vi "test_AllCodeInCorrectLVVersion.vi"() -> (3 "Pass?":bool)   [LabVIEW 2019, in "Tests.General.lvlib"]
uses:
  Tests.General.lvlib
panel:
  in  "LV version":string="19.0"
  out "Failed results":cluster{"file":path, "FileLVVersion":string}[](array[cluster])
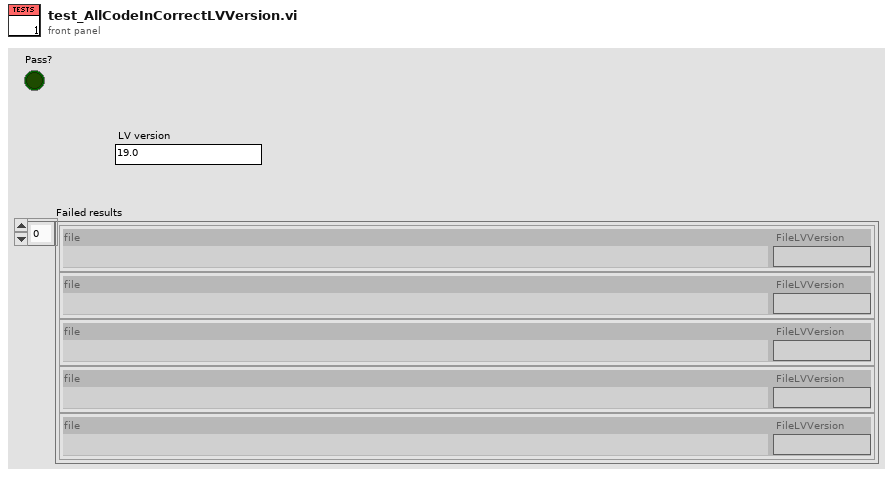
[diagram p1: front panel]
types:
  T1 = cluster{"dup file":path, "Project.GetFileLVVersion":string}
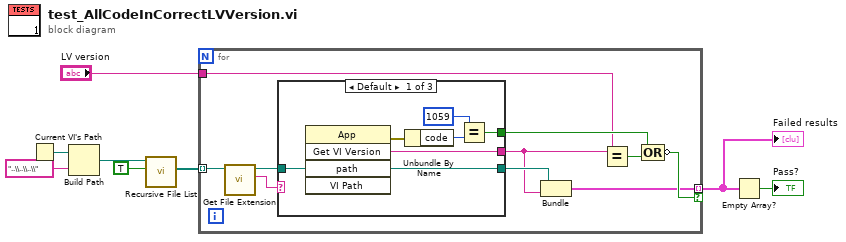
[diagram p0: block diagram]
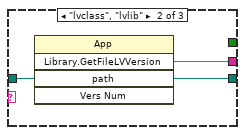
[diagram p2: hidden frame]
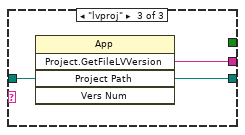
[diagram p3: hidden frame]
diagram:
  n1 = Current VI's Path() -> (path=w8:path)
  n2 = Build Path(base path=w8, name or relative path="..\\..\\..\\") -> (appended path=w6:path)
  n3 = call <vilib>:"Recursive File List.vi"("Treat LLBs as Folders?"=TRUE, "Folder Path"=w6) -> ("All Files in Dir"=w4:path[])  [unwired: 5 in, 4 out]
  n4 = for {
    tunnel: w4 -> [w18] mode=indexing
    tunnel: [w10] -> w3 mode=indexing if=w11
    tunnel: "LV version" -> [w9]
    n5 = call <vilib>:"Get File Extension.vi"("file"=w18) -> ("lowercase file extension"=w16:string, "dup file"=w17:path)  [unwired: 6 in, 3 out]
    n6 = case shown="Default" w16 {
      tunnel: w17 -> [w20 w25 w27]
      tunnel: [w24 w26 w28] -> w14
      tunnel: [w19 _ _] -> w12
      tunnel: [w20 w25 w27] -> w15
      frame Default {
        n7 = invoke class="App" method="Get VI Version"("path"=w20) -> (error out=w23:errorcluster, "GetVIVers"=w24:string)  [unwired: 4 in, 3 out]
        n8 = Unbundle By Name(w23) -> ("code"=w22:i32)
        n9 = Equal?(x=1059 ("code"), y=w22) -> (x = y?=w19:bool)
      }
      frame "lvclass", "lvlib" {
        n10 = invoke class="App" method="Library.GetFileLVVersion"("path"=w25) -> ("Library.GetFileLVVersion"=w26:string)  [unwired: 4 in, 4 out]
      }
      frame "lvproj" {
        n11 = invoke class="App" method="Project.GetFileLVVersion"("Project Path"=w27) -> ("Project.GetFileLVVersion"=w28:string)  [unwired: 4 in, 4 out]
      }
    }
    n12 = Bundle("dup file"=w15, "Project.GetFileLVVersion"=w14) -> (w10:T1)  [unwired: 1 in]
    n13 = Equal?(x=w14, y=w9) -> (x = y?=w13:bool)
    n14 = Compound Arithmetic op=OR(w12, w13) -> (invert w11:bool)
  }
  "Failed results" <- w3
  n15 = Empty Array?(array=w3) -> (empty?=→"Pass?":bool)
